vi "Begin.vi"(8 "error in":errorcluster, 10 "Two drivers?":bool) -> (0 "error out":errorcluster)   [LabVIEW 2018]
doc: "Called before other user functions, this VI is expected to open initial I/O refnums, load in file data, and do all program initialization. Notice that the <B>error out</B> terminal is simply used for data flow. Wiring it to other structures or subVIs ensures that this VI runs first."
uses:
  <vilib>/Rock Robotics/WPI/DriverStation/WPI_DriverStationRobotMode2.ctl
  Classes/Drive/Simulated Drive/Simulated Drive.lvclass
  C:/Users/Public/Documents/2019DeepSpace/Classes/Drive/Drive.lvclass
  Classes/Drive/Pod Drive/Pod Drive.lvclass
  Classes/Joysticks/One Driver/One Driver.lvclass
  C:/Users/Public/Documents/2019DeepSpace/Classes/Joysticks/Joysticks.lvclass
  TypeDefs/RobotObjects.ctl
  Classes/Drive/Drive.lvclass
  Classes/Pnematics control/Pneumatics.lvclass
  Classes/Vision/Vision.lvclass
  Classes/Joysticks/Joysticks.lvclass
  Classes/Elevator/Elevator.lvclass
  Classes/Hatch/Hatch.lvclass
  Classes/Cargo/Cargo.lvclass
  Classes/Elevator/Elevator Concrete/Elevator Concrete.lvclass
  C:/Users/Public/Documents/2019DeepSpace/Classes/Elevator/Elevator.lvclass
  Classes/Cargo/Cargo Concrete/Cargo Concrete.lvclass
  C:/Users/Public/Documents/2019DeepSpace/Classes/Cargo/Cargo.lvclass
  Classes/Pnematics control/TypeDefs/Solenoids.ctl
  Classes/Pnematics control/Solenoids/Solenoids.lvclass
  Classes/Pnematics control/Solenoids/DoubleSolenoid.lvclass
  C:/Users/Public/Documents/2019DeepSpace/Classes/Pnematics control/Solenoids/Solenoids.lvclass
  Classes/Cargo/Cargo Simulated/Cargo Simulated.lvclass
  Classes/Elevator/Elevator Simulated/Elevator Simulated.lvclass
  Classes/Hatch/Hatch Concrete/Hatch Concrete.lvclass
  C:/Users/Public/Documents/2019DeepSpace/Classes/Hatch/Hatch.lvclass
  Classes/Hatch/Hatch Simulated/Hatch Simulated.lvclass
  Classes/Config/FileConfig/FileConfig.lvclass
  C:/Users/Public/Documents/2019DeepSpace/Classes/Config/Config.lvclass
  Classes/Joysticks/Two Drivers/Two Drivers.lvclass
  Classes/Config/Config.lvclass
  Classes/Drive/Controls/Drive Sensor Data.ctl
  Classes/Drive/Controls/Motion Magic Constants.ctl
  Classes/Elevator/Controls/Elevator IDs.ctl
  Classes/Elevator/Controls/Elevator Constants.ctl
  Classes/Elevator/Controls/Elevator Position.ctl
  Classes/Elevator/Controls/Arm Position Values.ctl
  Classes/Joysticks/Joysticks.lvclass/Joysticks.ctl
  Classes/Drive/Drive.lvclass/Drive.ctl
  Classes/Elevator/Elevator.lvclass/Elevator.ctl
  Classes/Joysticks/Public Methods/Write Sensitivity(x).vi
  Classes/Joysticks/Public Methods/Write Sensitivity(y).vi
  Classes/Drive/Public Methods/Write Drive Velocity Low Gear.vi
  Classes/Drive/Public Methods/Write Drive Velocity High Gear.vi
  Classes/Drive/Public Methods/Write Drive Motion Magic Primary Low Gear.vi
  Classes/Drive/Public Methods/Write Drive Motion Magic Primary High Gear.vi
  Classes/Drive/Public Methods/Write Drive Motion Magic Secondary High Gear.vi
  Classes/Drive/Public Methods/Write Drive Motion Magic Secondary Low Gear.vi
  Classes/Drive/Public Methods/Write Motion Magic Constants.vi
  Classes/Elevator/Public Methods/Write Arm Position Values.vi
  Robot Global Data.vi
  RobotGlobal.vi
panel:
  out "Config File Not Found or Error":bool
  in  "Bypass File Reading and use Defaults?":bool
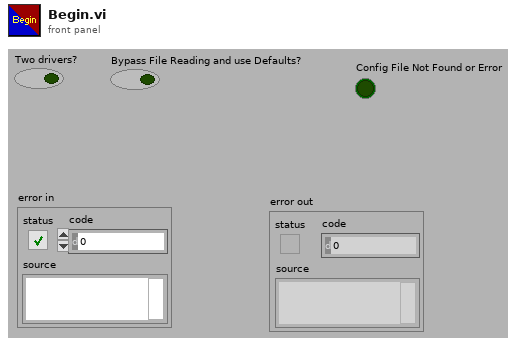
[diagram p1: front panel]
types:
  T1 = typedef "WPI_DriverStationRobotMode2.ctl" = enum16{"Autonomous Disabled", "Autonomous Enabled", "Teleop Disabled", "Teleop Enabled", "Disconnected", "Finish", "Test Disabled", "Test Enabled", "Emergency Stopped"}
  T2 = typedef "Elevator.lvlib/Elevator.lvclass/Arm Position Values.ctl" = cluster{"C0 Arm":dbl, "C1 Arm":dbl, "C2 Arm":dbl, "H1 Arm":dbl, "H2 Arm":dbl, "C0 Wrist":dbl, "C1 Wrist ":dbl, "C2 Wrist":dbl, "H1 Wrist":dbl, "H2 Wrist":dbl, "Deploy Arm":dbl, "Deploy Wrist":dbl, "Climb Arm":dbl, "Climb Wrist":dbl, "Stowed Arm":dbl, "Stowed Wrist":dbl}
  T3 = typedef "Elevator.lvlib/Elevator.lvclass/Elevator Position.ctl" = enum16{"C0, Cargo Ground", "C1, LV1 Cargo", "C2, Cargo Ship Cargo", "H0, LV1 Hatch", "H1, LV2 Hatch"}
  T4 = typedef "Elevator.lvlib/Elevator.lvclass/Elevator Constants.ctl" = cluster{"Arm Motion Magic Max Velocity":u32, "Arm Motion Magic Max Acceleration":u32, "Wrist Motion Magic Max Velocity":u32, "Wrist Motion Magic Max Acceleration":u32, "Arm Gear Ratio":dbl, "Wrist Gear Ratio":dbl, "Arm Encoder ABS Value":i32, "Wrist Encoder ABS Value":i32}
  T5 = typedef "Elevator.lvlib/Elevator.lvclass/Elevator IDs.ctl" = cluster{"Wrist":u8, "Left Master":u8, "Left Slave":u8, "Right Master":u8, "Right Slave":u8, "Vacumm Pump 1":u8, "Vacumm Pump 2":u8}
  T6 = typedef "Drive.lvlib/Drive.lvclass/Motion Magic Constants.ctl" = cluster{"Low Gear Max Velocity":u32, "High Gear Max Velocity":u32, "Motion Magic Low Gear Max Velocity":u32, "Motion Magic Low Gear Max Acceleration":u32, "Motion Magic High Gear Max Velocity":u32, "Motion Magic High Gear Max Acceleration":u32}
  T7 = typedef "Drive.lvlib/Drive.lvclass/Drive Sensor Data.ctl" = cluster{"Drive Right Invert":bool, "Drive Right Sensor Phase":bool, "Drive Left Invert":bool, "Drive Left Sensor Phase":bool}
  T8 = typedef "Pneumatics control.lvlib/Pneumatics.lvclass/Solenoids.ctl" = cluster{"DriveShift":refnum<class "Solenoids.lvclass">, "ArmLock":refnum<class "Solenoids.lvclass">, "HatchArm":refnum<class "Solenoids.lvclass">, "HatchGrabber":refnum<class "Solenoids.lvclass">}
  T9 = typedef "RobotObjects.ctl" = cluster{"Drive.lvclass":refnum<class "Drive.lvclass">, "Pneumatics.lvclass":refnum<class "Pneumatics.lvclass">, "Vision.lvclass":refnum<class "Vision.lvclass">, "Joysticks.lvclass":refnum<class "Joysticks.lvclass">, "Elevator.lvclass":refnum<class "Elevator.lvclass">, "Hatch.lvclass":refnum<class "Hatch.lvclass">, "Cargo.lvclass":refnum<class "Cargo.lvclass">}
  T10 = typedef "Config.lvlib/Config.lvclass/Simulated Classes.ctl" = cluster{"Drive":bool, "Pneumatics":bool, "Cargo":bool, "Elevator":bool, "Hatch":bool}
  T11 = typedef "Config.lvlib/Config.lvclass/Drivetrain Data.ctl" = cluster{"Right":T12, "Left":T12, "Drive Velocity Low Gear":T13, "Drive Velocity High Gear":T13, "Drive Motion Magic Primary Low Gear":T13, "Drive Motion Magic Primary High Gear":T13, "Drive Motion Magic Secondary Low Gear":T13, "Drive Motion Magic Secondary High Gear":T13, "Drive Right Invert":bool, "Drive Right Sensor Phase":bool, "Drive Left Invert":bool, "Drive Left Sensor Phase":bool, "Low Gear Max Velocity":u32, "High Gear Max Velocity":u32, "Motion Magic Low Gear Max Velocity":u32, "Motion Magic Low Gear Max Acceleration":u32, "Motion Magic High Gear Max Velocity":u32, "Motion Magic High Gear Max Acceleration":u32}
  T12 = typedef "Drive.lvlib/Pod Drive.lvclass/Pod.ctl" = cluster{"Talon":u8, "Victor1":u8, "Victor2":u8}
  T13 = typedef "CTRE_Phoenix_MotorControl_SlotStructure.ctl" = cluster{"P":dbl, "I":dbl, "D":dbl, "F":dbl, "integralZone":dbl, "allowableClosedLoopError":i32, "maxIntegralAccumulator":dbl, "closedLoopPeakOutput":dbl, "closedLoopPeriod":i32}
  T14 = typedef "Config.lvlib/Config.lvclass/Elevator Data.ctl" = cluster{"Wrist":u8, "Left Master":u8, "Left Slave":u8, "Right Master":u8, "Right Slave":u8, "Elevator Wrist PID":T13, "Elevator Arm PID":T13, "Vacumm Pump 1":u8, "Vacumm Pump 2":u8, "Arm Motion Magic Max Velocity":u32, "Arm Motion Magic Max Acceleration":u32, "Wrist Motion Magic Max Velocity":u32, "Wrist Motion Magic Max Acceleration":u32, "Arm Gear Ratio":dbl, "Wrist Gear Ratio":dbl, "C0 Arm":dbl, "C1 Arm":dbl, "C2 Arm":dbl, "H1 Arm":dbl, "H2 Arm":dbl, "C0 Wrist":dbl, "C1 Wrist ":dbl, "C2 Wrist":dbl, "H1 Wrist":dbl, "H2 Wrist":dbl, "Deploy Arm":dbl, "Deploy Wrist":dbl, "Climb Arm":dbl, "Climb Wrist":dbl, "Arm Encoder ABS Value":i32, "Wrist Encoder ABS Value":i32}
  T15 = typedef "Config.lvlib/Config.lvclass/Pneumatics Data.ctl" = cluster{"PCM ID":u8, "Drive Shift Low Gear":T16, "Drive Shift High Gear":T16, "Hatch Grabber Release":T16, "Hatch Grabber Capture":T16, "Arm Lock Deploy":T16, "Arm Lock Retract":T16}
  T16 = typedef "WPI_SolenoidChannel.ctl" = enum8{"Solenoid 0", "Solenoid 1", "Solenoid 2", "Solenoid 3", "Solenoid 4", "Solenoid 5", "Solenoid 6", "Solenoid 7", "Invalid"}
  T17 = typedef "Config.lvlib/Config.lvclass/PWM Data.ctl" = cluster{"Cargo Intake Left":T18, "Cargo Intake Right":T18}
  T18 = typedef "FPGA_DIOPWMChannel.ctl" = enum8{"PWM 0", "PWM 1", "PWM 2", "PWM 3", "PWM 4", "PWM 5", "PWM 6", "PWM 7", "PWM 8", "PWM 9", "PWM MXP 0", "PWM MXP 1", "PWM MXP 2", "PWM MXP 3", "PWM MXP 4", "PWM MXP 5", "PWM MXP 6", "PWM MXP 7", "PWM MXP 8", "PWM MXP 9", "Invalid"}
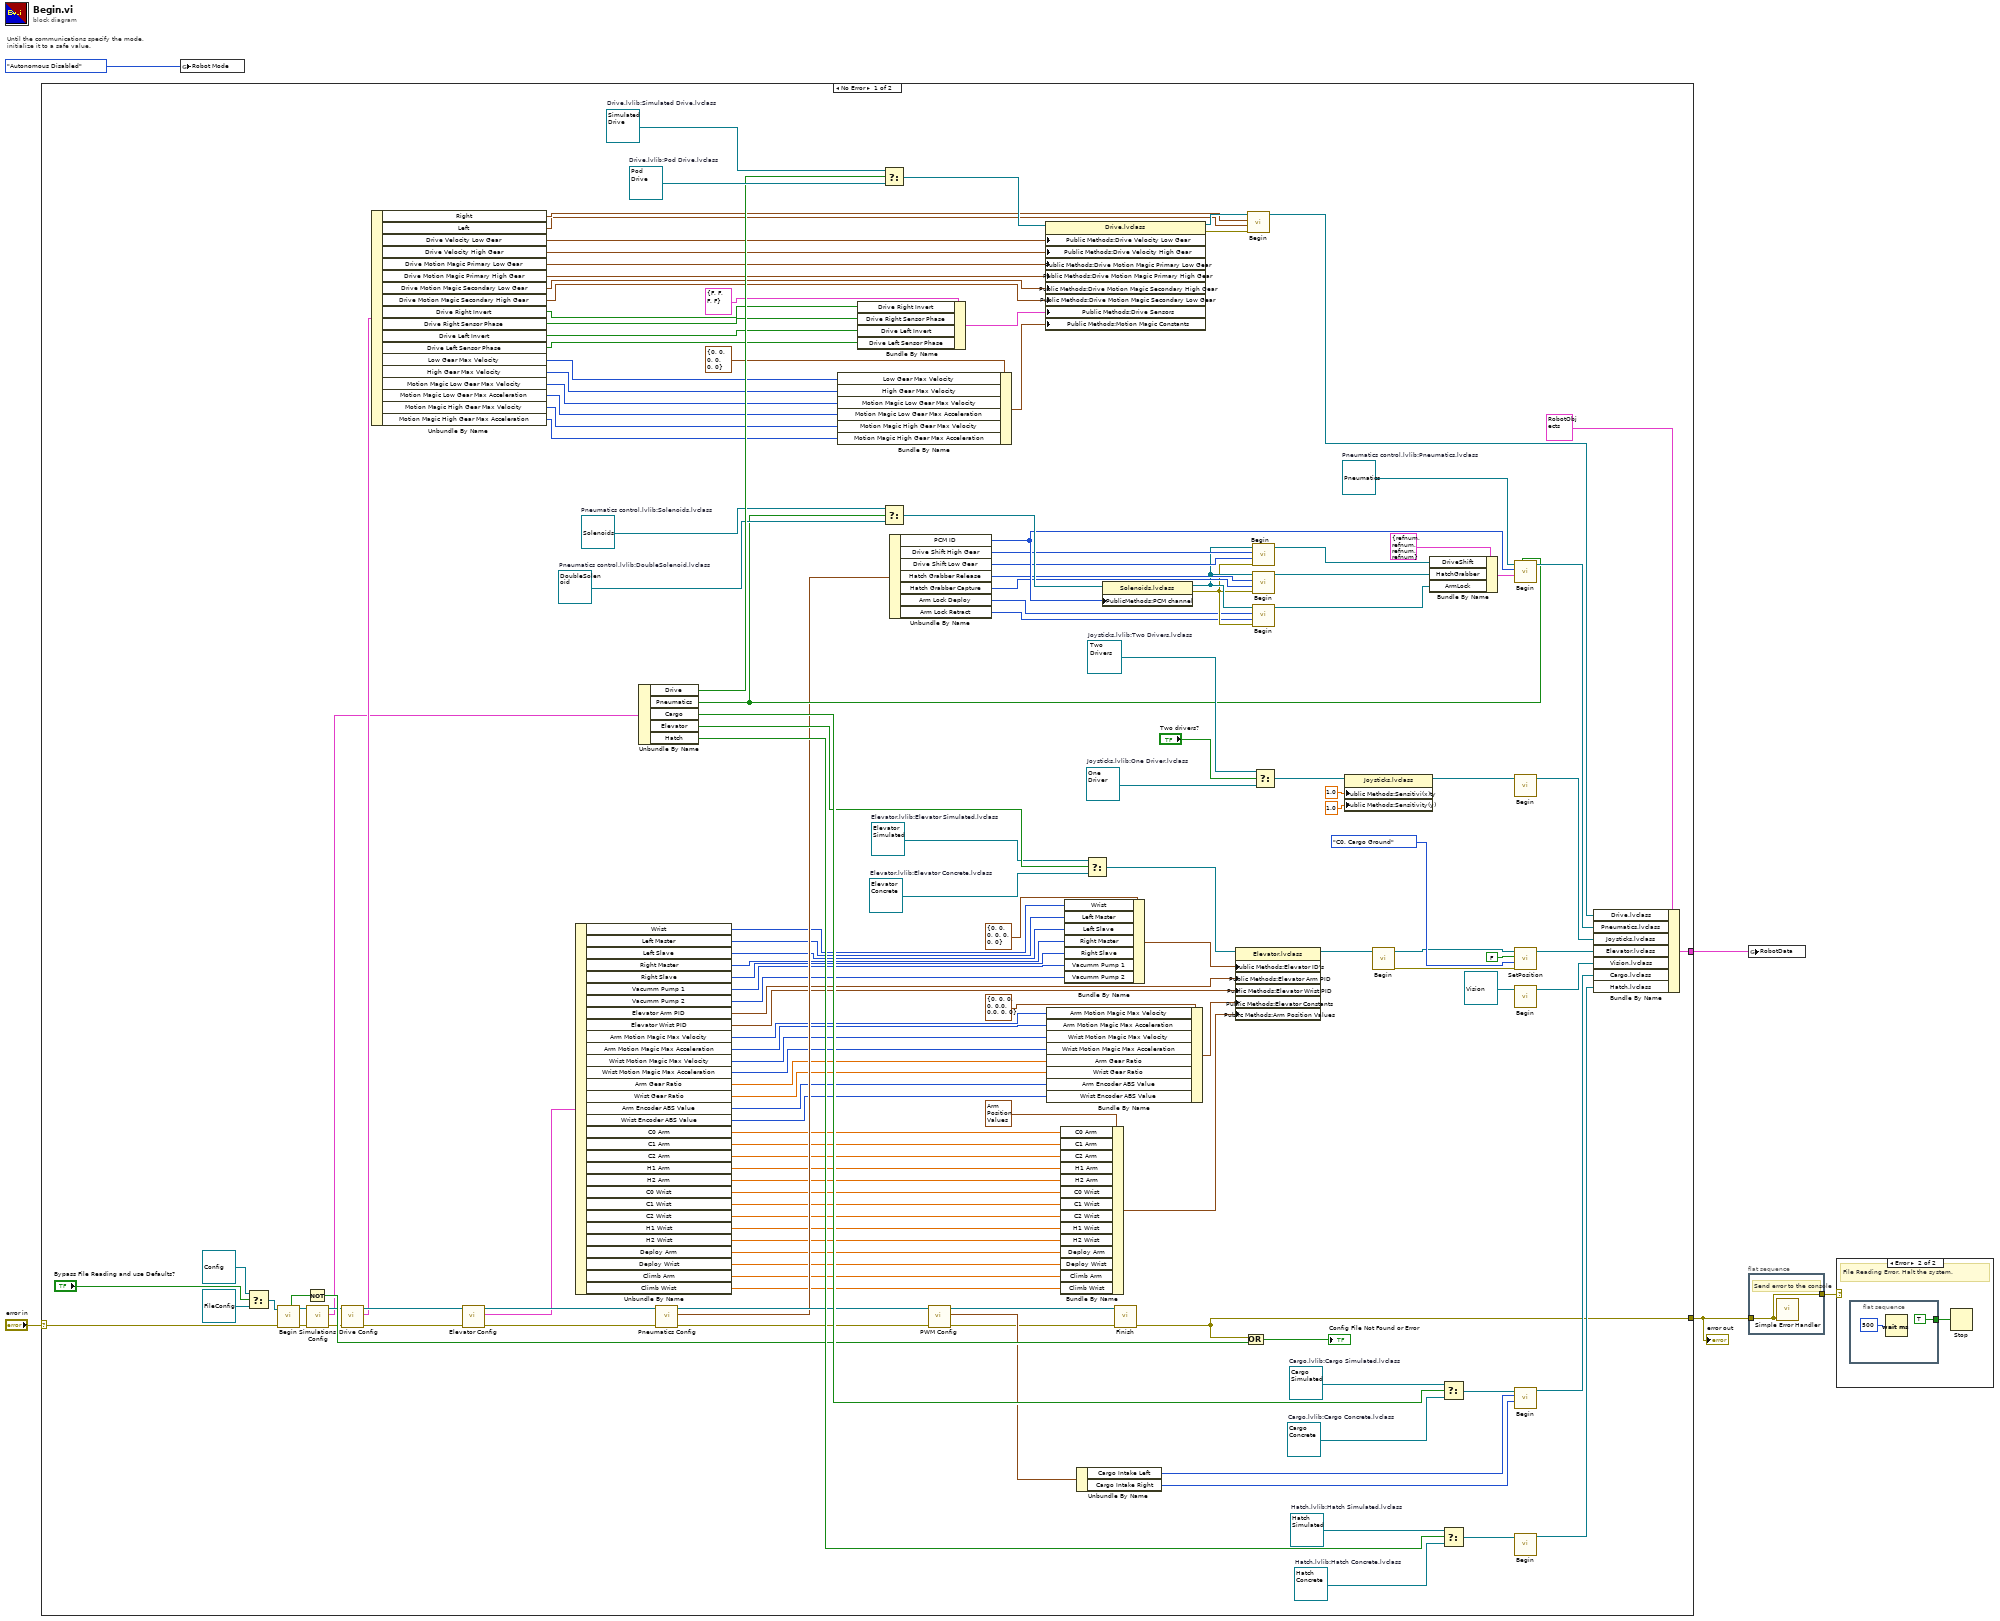
[diagram p0: block diagram]
diagram:
  # "Until the communications specify the mode,\ninitialize it to a safe value."
  n1 = case shown="No Error" "error in" {
    selector: "error in" -> [w85 w152]
    tunnel: [w148 _] -> w2
    tunnel: [w75 w152] -> w3
    frame No Error {
      w116 = refnum<class "Two Drivers.lvclass"> refnum  # Joysticks.lvlib:Two Drivers.lvclass
      w126 = refnum<class "Hatch Simulated.lvclass"> refnum  # Hatch.lvlib:Hatch Simulated.lvclass
      w125 = refnum<class "Hatch Concrete.lvclass"> refnum  # Hatch.lvlib:Hatch Concrete.lvclass
      w127 = refnum<class "Elevator Simulated.lvclass"> refnum  # Elevator.lvlib:Elevator Simulated.lvclass
      w130 = refnum<class "Cargo Simulated.lvclass"> refnum  # Cargo.lvlib:Cargo Simulated.lvclass
      w139 = refnum<class "DoubleSolenoid.lvclass"> refnum  # Pneumatics control.lvlib:DoubleSolenoid.lvclass
      w138 = refnum<class "Solenoids.lvclass"> refnum  # Pneumatics control.lvlib:Solenoids.lvclass
      w143 = refnum<class "Pneumatics.lvclass"> refnum  # Pneumatics control.lvlib:Pneumatics.lvclass
      w132 = refnum<class "Cargo Concrete.lvclass"> refnum  # Cargo.lvlib:Cargo Concrete.lvclass
      w119 = refnum<class "Elevator Concrete.lvclass"> refnum  # Elevator.lvlib:Elevator Concrete.lvclass
      w118 = refnum<class "One Driver.lvclass"> refnum  # Joysticks.lvlib:One Driver.lvclass
      w149 = refnum<class "Pod Drive.lvclass"> refnum  # Drive.lvlib:Pod Drive.lvclass
      w151 = refnum<class "Simulated Drive.lvclass"> refnum  # Drive.lvlib:Simulated Drive.lvclass
      n2 = Select(t=refnum<class "Config.lvclass"> refnum ("Config.lvlib:Config.lvclass"), s="Bypass File Reading and use Defaults?", f=refnum<class "FileConfig.lvclass"> refnum ("Config.lvlib:FileConfig.lvclass")) -> (s? t:f=w111:refnum<class "Config.lvclass">)
      n3 = call-dynamic "Begin.vi"("error in (no error)"=w85, "Config in"=w111) -> ("error out"=w89:errorcluster, "Config out"=w59:refnum<class "Config.lvclass">, "File Found?"=w94:bool)  [unwired: 7 in]
      n4 = Not(x=w94) -> (.not. x?=w106:bool)
      n5 = call-dynamic "Simulations Config.vi"("error in (no error)"=w89, "Config in"=w59) -> ("error out"=w60:errorcluster, "Simulated Classes"=w57:T10, "Config out"=w58:refnum<class "Config.lvclass">)  [unwired: 6 in, 1 out]
      n6 = call-dynamic "Drive Config.vi"("error in (no error)"=w60, "Config in"=w58) -> ("error out"=w88:errorcluster, "Robot Drivetrain Data"=w105:T11, "Config out"=w109:refnum<class "Config.lvclass">)  [unwired: 4 in, 3 out]
      n7 = Unbundle By Name(w105) -> ("Right"=w91:T12, "Left"=w90:T12, "Drive Velocity Low Gear"=w74:T13, "Drive Velocity High Gear"=w73:T13, "Drive Motion Magic Primary Low Gear"=w72:T13, "Drive Motion Magic Primary High Gear"=w69:T13, "Drive Motion Magic Secondary Low Gear"=w70:T13, "Drive Motion Magic Secondary High Gear"=w71:T13, "Drive Right Invert"=w79:bool, "Drive Right Sensor Phase"=w81:bool, "Drive Left Invert"=w82:bool, "Drive Left Sensor Phase"=w83:bool, "Low Gear Max Velocity"=w61:u32, "High Gear Max Velocity"=w62:u32, "Motion Magic Low Gear Max Velocity"=w63:u32, "Motion Magic Low Gear Max Acceleration"=w64:u32, "Motion Magic High Gear Max Velocity"=w65:u32, "Motion Magic High Gear Max Acceleration"=w66:u32)
      n8 = call-dynamic "Elevator Config.vi"("error in (no error)"=w88, "Config in"=w109) -> ("error out"=w87:errorcluster, "Elevator Data"=w104:T14, "Config out"=w108:refnum<class "Config.lvclass">)  [unwired: 4 in, 3 out]
      n9 = Unbundle By Name(w104) -> ("Wrist"=w53:u8, "Left Master"=w52:u8, "Left Slave"=w51:u8, "Right Master"=w50:u8, "Right Slave"=w49:u8, "Vacumm Pump 1"=w48:u8, "Vacumm Pump 2"=w47:u8, "Elevator Arm PID"=w46:T13, "Elevator Wrist PID"=w45:T13, "Arm Motion Magic Max Velocity"=w42:u32, "Arm Motion Magic Max Acceleration"=w41:u32, "Wrist Motion Magic Max Velocity"=w40:u32, "Wrist Motion Magic Max Acceleration"=w39:u32, "Arm Gear Ratio"=w28:dbl, "Wrist Gear Ratio"=w27:dbl, "Arm Encoder ABS Value"=w10:i32, "Wrist Encoder ABS Value"=w9:i32, "C0 Arm"=w25:dbl, "C1 Arm"=w24:dbl, "C2 Arm"=w23:dbl, "H1 Arm"=w22:dbl, "H2 Arm"=w21:dbl, "C0 Wrist"=w20:dbl, "C1 Wrist"=w19:dbl, "C2 Wrist"=w18:dbl, "H1 Wrist"=w17:dbl, "H2 Wrist"=w16:dbl, "Deploy Arm"=w15:dbl, "Deploy Wrist"=w14:dbl, "Climb Arm"=w13:dbl, "Climb Wrist"=w12:dbl)
      n10 = Unbundle By Name(w57) -> ("Drive"=w144:bool, "Pneumatics"=w114:bool, "Cargo"=w129:bool, "Elevator"=w128:bool, "Hatch"=w124:bool)
      n11 = call-dynamic "Pneumatics Config.vi"("error in (no error)"=w87, "Config in"=w108) -> ("error out"=w86:errorcluster, "Pneumatics Data"=w103:T15, "Config out"=w107:refnum<class "Config.lvclass">)  [unwired: 5 in, 2 out]
      n12 = Bundle By Name(cluster=T6 {"Low Gear Max Velocity"=0, "High Gear Max Velocity"=0, "Motion Magic Low Gear Max Velocity"=0, "Motion Magic Low Gear Max Acceleration"=0, "Motion Magic High Gear Max Velocity"=0, "Motion Magic High Gear Max Acceleration"=0} ("Motion Magic Constants"), "Low Gear Max Velocity"=w61, "High Gear Max Velocity"=w62, "Motion Magic Low Gear Max Velocity"=w63, "Motion Magic Low Gear Max Acceleration"=w64, "Motion Magic High Gear Max Velocity"=w65, "Motion Magic High Gear Max Acceleration"=w66) -> (w67:T6)
      n13 = Bundle By Name(cluster=T7 {"Drive Right Invert"=FALSE, "Drive Right Sensor Phase"=FALSE, "Drive Left Invert"=FALSE, "Drive Left Sensor Phase"=FALSE} ("Drive Sensors"), "Drive Right Invert"=w79, "Drive Right Sensor Phase"=w81, "Drive Left Invert"=w82, "Drive Left Sensor Phase"=w83) -> (w80:T7)
      n14 = Select(t=w151, s=w144, f=w149) -> (s? t:f=w150:refnum<class "Drive.lvclass">)
      n15 = Select(t=w138, s=w114, f=w139) -> (s? t:f=w137:refnum<class "Solenoids.lvclass">)
      n16 = Unbundle By Name(w103) -> ("PCM ID"=w101:u8, "Drive Shift High Gear"=w100:T16, "Drive Shift Low Gear"=w99:T16, "Hatch Grabber Release"=w98:T16, "Hatch Grabber Capture"=w97:T16, "Arm Lock Deploy"=w35:T16, "Arm Lock Retract"=w34:T16)
      n17 = call-dynamic "PWM Config.vi"("error in (no error)"=w86, "Config in"=w107) -> ("error out"=w78:errorcluster, "PWM Data"=w102:T17, "Config out"=w77:refnum<class "Config.lvclass">)  [unwired: 5 in, 2 out]
      n18 = property class="Drive.lvclass"(reference=w150, "Public Methods:Drive Velocity Low Gear"=w74, "Public Methods:Drive Velocity High Gear"=w73, "Public Methods:Drive Motion Magic Primary Low Gear"=w72, "Public Methods:Drive Motion Magic Primary High Gear"=w69, "Public Methods:Drive Motion Magic Secondary High Gear"=w70, "Public Methods:Drive Motion Magic Secondary Low Gear"=w71, "Public Methods:Drive Sensors"=w80, "Public Methods:Motion Magic Constants"=w67) -> (reference out=w93:refnum<class "Drive.lvclass">, error out=w92:errorcluster)  [unwired: 1 in]
      n19 = Bundle By Name(cluster=T4 {"Arm Motion Magic Max Velocity"=0, "Arm Motion Magic Max Acceleration"=0, "Wrist Motion Magic Max Velocity"=0, "Wrist Motion Magic Max Acceleration"=0, "Arm Gear Ratio"=0.0, "Wrist Gear Ratio"=0.0, "Arm Encoder ABS Value"=0, "Wrist Encoder ABS Value"=0} ("Elevator Constants"), "Arm Motion Magic Max Velocity"=w42, "Arm Motion Magic Max Acceleration"=w41, "Wrist Motion Magic Max Velocity"=w40, "Wrist Motion Magic Max Acceleration"=w39, "Arm Gear Ratio"=w28, "Wrist Gear Ratio"=w27, "Arm Encoder ABS Value"=w10, "Wrist Encoder ABS Value"=w9) -> (w43:T4)
      n20 = Bundle By Name(cluster=T2 {"C0 Arm"=0.0, "C1 Arm"=0.0, "C2 Arm"=0.0, "H1 Arm"=0.0, "H2 Arm"=0.0, "C0 Wrist"=0.0, "C1 Wrist "=0.0, "C2 Wrist"=0.0, "H1 Wrist"=0.0, "H2 Wrist"=0.0, "Deploy Arm"=0.0, "Deploy Wrist"=0.0, "Climb Arm"=0.0, "Climb Wrist"=0.0, "Stowed Arm"=0.0, "Stowed Wrist"=0.0} ("input cluster"), "C0 Arm"=w25, "C1 Arm"=w24, "C2 Arm"=w23, "H1 Arm"=w22, "H2 Arm"=w21, "C0 Wrist"=w20, "C1 Wrist"=w19, "C2 Wrist"=w18, "H1 Wrist"=w17, "H2 Wrist"=w16, "Deploy Arm"=w15, "Deploy Wrist"=w14, "Climb Arm"=w13, "Climb Wrist"=w12) -> (w11:T2)
      n21 = Bundle By Name(cluster=T5 {"Wrist"=0, "Left Master"=0, "Left Slave"=0, "Right Master"=0, "Right Slave"=0, "Vacumm Pump 1"=0, "Vacumm Pump 2"=0} ("Elevator ID's"), "Wrist"=w53, "Left Master"=w52, "Left Slave"=w51, "Right Master"=w50, "Right Slave"=w49, "Vacumm Pump 1"=w48, "Vacumm Pump 2"=w47) -> (w55:T5)
      n22 = Unbundle By Name(w102) -> ("Cargo Intake Left"=w96:T18, "Cargo Intake Right"=w95:T18)
      n23 = Select(t=w127, s=w128, f=w119) -> (s? t:f=w120:refnum<class "Elevator.lvclass">)
      n24 = property class="Solenoids.lvclass"(reference=w137, "PublicMethods:PCM channel"=w101) -> (reference out=w37:refnum<class "Solenoids.lvclass">, error out=w36:errorcluster)  [unwired: 1 in]
      n25 = call-dynamic "Finish.vi"("error in (no error)"=w78, "Config in"=w77) -> ("error out"=w75:errorcluster)  [unwired: 8 in, 1 out]
      n26 = property class="Elevator.lvclass"(reference=w120, "Public Methods:Elevator ID's"=w55, "Public Methods:Elevator Arm PID"=w46, "Public Methods:Elevator Wrist PID"=w45, "Public Methods:Elevator Constants"=w43, "Public Methods:Arm Position Values"=w11) -> (reference out=w56:refnum<class "Elevator.lvclass">)  [unwired: 1 in, 1 out]
      n27 = Or(x=w75, y=w106) -> (x .or. y?=→"Config File Not Found or Error":bool)
      n28 = call-dynamic "Begin.vi"("error in (no error)"=w92, "Left"=w90, "Right"=w91, "Drive in"=w93) -> ("Drive out"=w147:refnum<class "Drive.lvclass">)  [unwired: 6 in, 1 out]
      n29 = call-dynamic "Begin.vi"("error in (no error)"=w36, "Reverse solenoid channel"=w99, "Forward Solenoid Channel"=w100, "Solenoids in"=w37) -> ("Solenoids out"=w136:refnum<class "Solenoids.lvclass">)  [unwired: 6 in, 1 out]
      n30 = call-dynamic "Begin.vi"("error in (no error)"=w36, "Reverse solenoid channel"=w97, "Forward Solenoid Channel"=w98, "Solenoids in"=w37) -> ("Solenoids out"=w135:refnum<class "Solenoids.lvclass">)  [unwired: 6 in, 1 out]
      n31 = call-dynamic "Begin.vi"("error in (no error)"=w36, "Reverse solenoid channel"=w34, "Forward Solenoid Channel"=w35, "Solenoids in"=w37) -> ("Solenoids out"=w38:refnum<class "Solenoids.lvclass">)  [unwired: 6 in, 1 out]
      n32 = Select(t=w116, s="Two drivers?", f=w118) -> (s? t:f=w117:refnum<class "Joysticks.lvclass">)
      n33 = property class="Joysticks.lvclass"(reference=w117, "Public Methods:Sensitivi(x)ty"=1.0 ("Sensitivi(x)ty"), "Public Methods:Sensitivity(y)"=1.0 ("Sensitivity(y)")) -> (reference out=w8:refnum<class "Joysticks.lvclass">)  [unwired: 1 in, 1 out]
      n34 = call-dynamic "Begin.vi"("Elevator in"=w56) -> ("error out"=w32:errorcluster, "Elevator out"=w31:refnum<class "Elevator.lvclass">)  [unwired: 9 in]
      n35 = Bundle By Name(cluster=T8 {"DriveShift"=refnum, "ArmLock"=refnum, "HatchArm"=refnum, "HatchGrabber"=refnum} ("Solenoids"), "DriveShift"=w136, "HatchGrabber"=w135, "ArmLock"=w38) -> (w140:T8)
      n36 = Select(t=w130, s=w129, f=w132) -> (s? t:f=w131:refnum<class "Cargo.lvclass">)
      n37 = Select(t=w126, s=w124, f=w125) -> (s? t:f=w123:refnum<class "Hatch.lvclass">)
      n38 = call-dynamic "Begin.vi"("Simulated?"=w114, "Solenoids"=w140, "Pneumatics Control Module (9)"=w101, "Pneumatics in"=w143) -> ("Pneumatics out"=w142:refnum<class "Pneumatics.lvclass">)  [unwired: 6 in, 1 out]
      n39 = call-dynamic "Begin.vi"("Joysticks in"=w8) -> ("Joysticks out"=w146:refnum<class "Joysticks.lvclass">)  [unwired: 9 in, 1 out]
      n40 = call-dynamic "SetPosition.vi"("error in (no error)"=w32, "Position"=Elevator_Position."C0, Cargo Ground", "Hach Grabed?"=FALSE, "Elevator in"=w31) -> ("Elevator out"=w30:refnum<class "Elevator.lvclass">)  [unwired: 6 in, 1 out]
      n41 = call-dynamic "Begin.vi"("Vision in"=refnum<class "Vision.lvclass"> refnum ("Vision.lvlib:Vision.lvclass")) -> ("Vision out"=w121:refnum<class "Vision.lvclass">)  [unwired: 9 in, 1 out]
      n42 = call-dynamic "Begin.vi"("Intake Right Channel"=w95, "Intake Left Channel"=w96, "Cargo in"=w131) -> ("Cargo out"=w133:refnum<class "Cargo.lvclass">)  [unwired: 7 in, 1 out]
      n43 = call-dynamic "Begin.vi"("Hatch in"=w123) -> ("Hatch out"=w122:refnum<class "Hatch.lvclass">)  [unwired: 9 in, 1 out]
      n44 = Bundle By Name(cluster=T9 {"Drive.lvclass"=refnum, "Pneumatics.lvclass"=refnum, "Vision.lvclass"=refnum, "Joysticks.lvclass"=refnum, "Elevator.lvclass"=refnum, "Hatch.lvclass"=refnum, "Cargo.lvclass"=refnum}, "Drive.lvclass"=w147, "Pneumatics.lvclass"=w142, "Joysticks.lvclass"=w146, "Elevator.lvclass"=w30, "Vision.lvclass"=w121, "Cargo.lvclass"=w133, "Hatch.lvclass"=w122) -> (w148:T9)
    }
    frame Error {
    }
  }
  "error out" <- w3
  n45 = global write "Robot Global Data.vi" "Robot Mode"(WPI_DriverStationRobotMode2."Autonomous Disabled" ("Robot Mode")) -> ()
  n46 = global write "RobotGlobal.vi" "RobotData"(w2) -> ()
  n47 = flat-sequence {
    tunnel: w3 -> [w153]
    tunnel: [w153] -> w1
    frame #0 {
      # "Send error to the console"
      n48 = call <vilib>:"Simple Error Handler.vi"("error in (no error)"=w153) -> ()  [unwired: 4 in, 5 out]
    }
  }
  n49 = case shown="Error" w1 {
    frame No Error {
    }
    frame Error {
      # "File Reading Error. Halt the system."
      n50 = flat-sequence {
        tunnel: [TRUE ("stop? (T)")] -> w154
        frame #0 {
          n51 = Wait (ms)(milliseconds to wait=u32 500) -> ()  [unwired: 1 out]
        }
      }
      n52 = Stop(stop? (T)=w154) -> ()
    }
  }
